vi "FindLatestRuntime_LocalDirectory.vi"(6 "error in":errorcluster, 9 "Path":path) -> (0 "error out":errorcluster, 1 "Found":bool, 3 "local runtime path":path, 4 "Version":T1)   [LabVIEW 2014, in "Raspberry Pi Compatible Compiler for LabVIEW.lvlib"]
uses:
  RasPi_Services/Download/RuntimeVersion.ctl
  Raspberry Pi Compatible Compiler for LabVIEW.lvlib
  RasPi_Services/Download/RasPiDownloader.lvlib
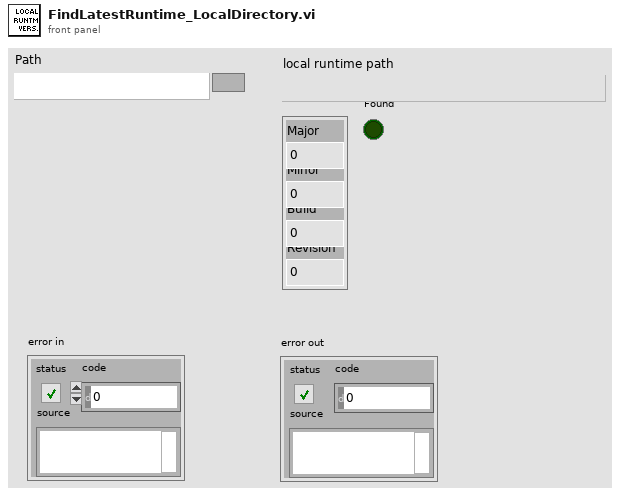
[diagram p1: front panel]
types:
  T1 = typedef "Raspberry Pi Compatible Compiler for LabVIEW.lvlib/RasPiDownloader.lvlib/RuntimeVersion.ctl" = cluster{"Major":i32, "Minor":i32, "Build":i32, "Revision":i32}
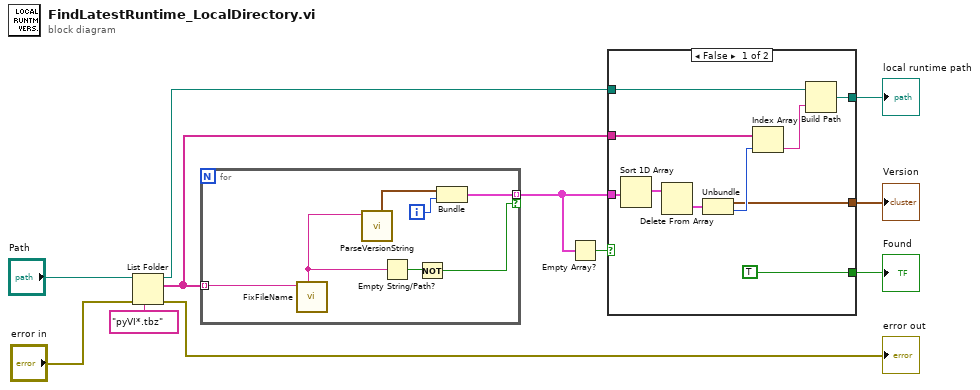
[diagram p0: block diagram]
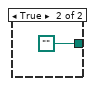
[diagram p2: hidden frame]
diagram:
  n1 = List Folder(path="Path", pattern="pyVI*.tbz", error in="error in") -> (path out=w3:path, filenames=w6:string[], error out=→"error out":errorcluster)  [unwired: 1 in, 1 out]
  n2 = for {
    tunnel: w6 -> [w12] mode=indexing
    tunnel: [w17] -> w7 mode=indexing if=w15
    i -> [w13]
    n3 = call "FixFileName.vi"("Filename"=w12) -> ("version"=w18:string)  [unwired: 7 in, 1 out]
    n4 = call "ParseVersionString.vi"("version string"=w18) -> ("Version"=w14:T1)  [unwired: 7 in, 1 out]
    n5 = Empty String/Path?(string/path=w18) -> (empty?=w16:bool)
    n6 = Not(x=w16) -> (.not. x?=w15:bool)
    n7 = Bundle("Version"=w14, w13) -> (w17:cluster{"Version":T1, i32})  [unwired: 1 in]
  }
  n8 = Empty Array?(array=w7) -> (empty?=w8:bool)
  n9 = case shown="False" w8 {
    tunnel: w7 -> [w28 _]
    tunnel: w6 -> [w25 _]
    tunnel: [TRUE _] -> w4
    tunnel: [w22 _] -> w5
    tunnel: w3 -> [w20 _]
    tunnel: [w19 path ""] -> w2
    frame False {
      n10 = Sort 1D Array(array=w28) -> (sorted array=w27:cluster{"Version":T1, i32}[])
      n11 = Delete From Array(array=w27) -> (deleted portion=w26:cluster{"Version":T1, i32})  [unwired: 2 in, 1 out]
      n12 = Unbundle(w26) -> ("Version"=w22:T1, w24:i32)
      n13 = Index Array(array=w25, index=w24) -> (element=w21:string)
      n14 = Build Path(base path=w20, name or relative path=w21) -> (appended path=w19:path)
    }
    frame True {
    }
  }
  "Found" <- w4
  "Version" <- w5
  "local runtime path" <- w2
